vi "After Launch Init Core.vi"(8 "error in (no error)":errorcluster, 11 "BNT_DAQmx-MCSV-Ctr2Freq in":refnum<class "BNT_DAQmx-MCSV-Ctr2Freq.lvclass">) -> (0 "error out":errorcluster, 3 "BNT_DAQmx-MCSV-Ctr2Freq out":refnum<class "BNT_DAQmx-MCSV-Ctr2Freq.lvclass">)   [LabVIEW 2017, in "BNT_DAQmx.lvlib" / "BNT_DAQmx-MCSV-Ctr2Freq.lvclass"]
doc: "Use <b>Pre Launch init.vi</b> method for sanity checks that are supposed to prevent the actor from launching if they fail. Use <B>this</B> method instead to initialize this actor when it has been activated. A corresponding high priority message will become dispatched before the <B>Actor Core.vi</b> is called.\n\n<b>Derived classed should call the parent methode first</b> and their own initialization code after.\n\nRefer also to the ongoing discussion at https://decibel.ni.com/content/message/57394#57394."
uses:
  BNT_DAQmx-MCSV-Ctr2Freq.lvclass
  BNT_DAQmx-MCSV-Ctr2Freq.lvclass/BNT_DAQmx-MCSV-Ctr2Freq.ctl
  BNT_DAQmx-MCSV/BNT_DAQmx-MCSV.lvclass
  CSPP_Core/Libraries/Utilities/CS++Utilities.lvlib
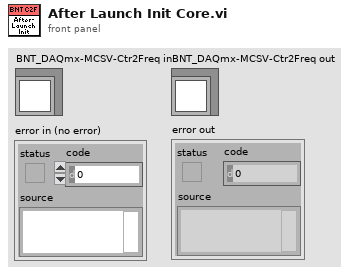
[diagram p1: front panel]
types:
  T1 = cluster{"Write Access":enum8{"Allowed", "Required", "None"}, "Read Access":enum8{"Allowed", "Required", "None"}}
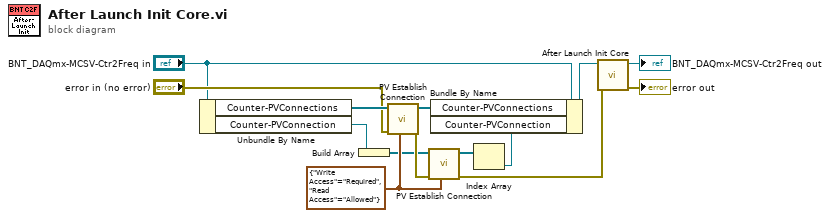
[diagram p0: block diagram]
diagram:
  w12 = T1 {"Write Access"=enum."Required", "Read Access"=enum."Allowed"} ("Access")
  n1 = Unbundle By Name("BNT_DAQmx-MCSV-Ctr2Freq in") -> ("Counter-PVConnections"=w7:refnum<class "PVConnection.lvclass">[], "Counter-PVConnection"=w10:refnum<class "PVConnection.lvclass">)
  n2 = Build Array(w10) -> (w9:refnum<class "PVConnection.lvclass">[])
  n3 = call "PV Establish Connection.vi"("Access (R/W allowed)"=w12, "Error In"="error in (no error)", "PVConnections in"=w7) -> ("Error Out"=w11:errorcluster, "PVConnections out"=w2:refnum<class "PVConnection.lvclass">[])  [unwired: 7 in]
  n4 = call "PV Establish Connection.vi"("Access (R/W allowed)"=w12, "Error In"=w11, "PVConnections in"=w9) -> ("Error Out"=w5:errorcluster, "PVConnections out"=w8:refnum<class "PVConnection.lvclass">[])  [unwired: 7 in]
  n5 = Index Array(array=w8) -> (element=w1:refnum<class "PVConnection.lvclass">)  [unwired: 1 in]
  n6 = Bundle By Name(cluster="BNT_DAQmx-MCSV-Ctr2Freq in", "Counter-PVConnections"=w2, "Counter-PVConnection"=w1) -> (w3:refnum<class "BNT_DAQmx-MCSV-Ctr2Freq.lvclass">)
  n7 = call-parent "After Launch Init Core.vi"("error in (no error)"=w5, "BNT_DAQmx-MCSV in"=w3) -> ("error out"=→"error out":errorcluster, "BNT_DAQmx-MCSV out"=→"BNT_DAQmx-MCSV-Ctr2Freq out":refnum<class "BNT_DAQmx-MCSV-Ctr2Freq.lvclass">)  [unwired: 8 in]
